vi "Host_DATAALL.vi"() -> ()   [LabVIEW 2017]
panel:
  out "Name array":string[](array[string])
  in  "All Data":string[][](array[string])
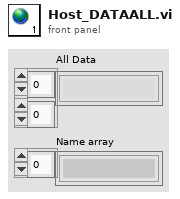
[diagram p1: front panel]
diagram:
